vi "Referencje Mem FVG.vi"(7 "Akcja (GET)":T1, 8 "AI wskazniki array in":refnum<vi>[](array[refnum]), 9 "DI wartosci array in":refnum<vi>[](array[refnum]), 10 "AI aktywne array in":refnum<vi>[](array[refnum]), 11 "AI_param array in":refnum<vi>[](array[refnum])) -> (0 "AI wskazniki array out":refnum<vi>[](array[refnum]), 1 "DI wartosci array out":refnum<vi>[](array[refnum]), 2 "AI aktywne array out":refnum<vi>[](array[refnum]), 3 "AI_param array out":refnum<vi>[](array[refnum]))   [LabVIEW 2014]
uses:
  Kontrolki/FVGs/Referencje Mem akcje.ctl
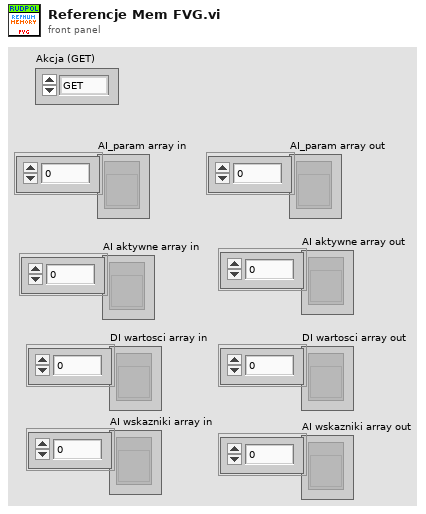
[diagram p1: front panel]
types:
  T1 = typedef "Referencje Mem akcje.ctl" = enum16{"GET", "SET"}
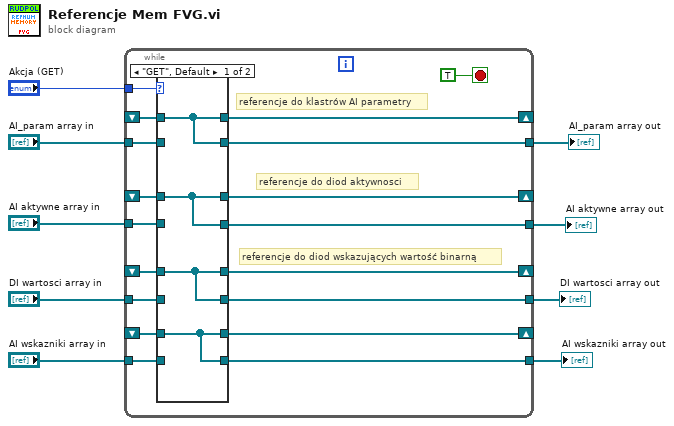
[diagram p0: block diagram]
diagram:
  n1 = while {
    tunnel: "AI_param array in" -> [w26]
    shift-right: [w27] -> _
    shift-left: _ -> [w25]
    tunnel: [w24] -> w8
    tunnel: "AI aktywne array in" -> [w22]
    tunnel: [w21] -> w6
    shift-right: [w20] -> _
    shift-left: _ -> [w19]
    tunnel: "DI wartosci array in" -> [w18]
    tunnel: [w17] -> w4
    shift-right: [w16] -> _
    shift-left: _ -> [w15]
    tunnel: [w14] -> w3
    tunnel: "AI wskazniki array in" -> [w13]
    shift-right: [w12] -> _
    shift-left: _ -> [w11]
    tunnel: "Akcja (GET)" -> [w10]
    stop <- TRUE stop-if-true
    # "referencje do diod wskazujących wartość binarną"
    # "referencje do diod aktywnosci"
    # "referencje do klastrów AI parametry"
    n2 = case shown="\"GET\", Default" w10 {
      tunnel: [w31 w35] -> w27
      tunnel: w26 -> [_ w35]
      tunnel: w25 -> [w31 _]
      tunnel: [w31 w35] -> w24
      tunnel: [w30 w34] -> w21
      tunnel: w22 -> [_ w34]
      tunnel: [w30 w34] -> w20
      tunnel: w19 -> [w30 _]
      tunnel: w18 -> [_ w33]
      tunnel: [w29 w33] -> w17
      tunnel: [w29 w33] -> w16
      tunnel: w15 -> [w29 _]
      tunnel: [w28 w32] -> w14
      tunnel: w13 -> [_ w32]
      tunnel: [w28 w32] -> w12
      tunnel: w11 -> [w28 _]
      frame "GET", Default {
      }
      frame "SET" {
      }
    }
  }
  "AI_param array out" <- w8
  "AI aktywne array out" <- w6
  "DI wartosci array out" <- w4
  "AI wskazniki array out" <- w3
